vi "Write To Csv.vi"(0 "File Path":path, 5 "StringArray":string[](array[string]), 7 "delimiter (Tab)":string, 11 "error in (no error)":errorcluster) -> (4 "String Out":string, 15 "error out":errorcluster)   [LabVIEW 2021, in "CustomSortPath.lvlib"]
doc: "This vi gets the file path , string array and delimiter as input. Writes the data into a .csv file."
uses:
  CustomSortPath.lvlib
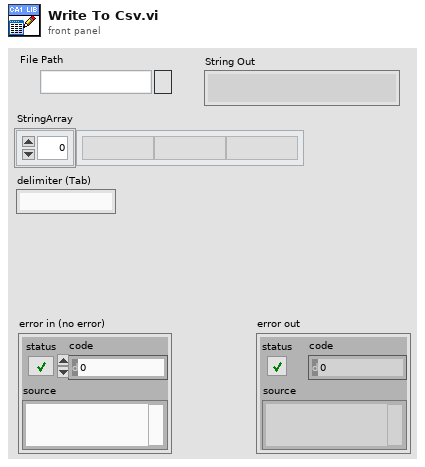
[diagram p1: front panel]
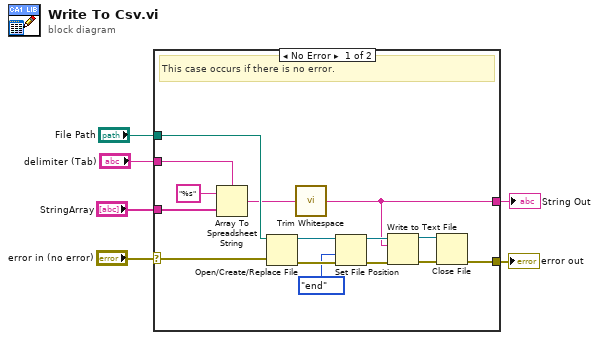
[diagram p0: block diagram]
diagram:
  n1 = case shown="No Error" "error in (no error)" {
    selector: "error in (no error)" -> [w9 w22]
    tunnel: "StringArray" -> [w20 _]
    tunnel: "delimiter (Tab)" -> [w19 _]
    tunnel: "File Path" -> [w18 _]
    tunnel: [w15 w22] -> w3
    tunnel: [w7 _] -> w1
    frame No Error {
      # "This case occurs if there is no error."
      n2 = Array To Spreadsheet String(delimiter (Tab)=w19, array=w20, 3:"%s" ("format string")) -> (spreadsheet string=w8:string)
      n3 = Open/Create/Replace File(file path (use dialog)=w18, error in=w9) -> (refnum out=w12:refnum<file>, error out=w14:errorcluster)  [unwired: 4 in, 1 out]
      n4 = call <vilib>:"Trim Whitespace.vi"("string"=w8) -> ("trimmed string"=w7:string)  [unwired: 1 in]
      n5 = Set File Position(refnum=w12, from (0:start)=enum16{"start", "end", "current"}."end", error in=w14) -> (refnum out=w10:refnum<file>, error out=w13:errorcluster)  [unwired: 1 in]
      n6 = Write to Text File(file (use dialog)=w10, text=w7, error in=w13) -> (refnum out=w16:refnum<file>, error out=w17:errorcluster)  [unwired: 1 in, 1 out]
      n7 = Close File(refnum=w16, error in=w17) -> (error out=w15:errorcluster)  [unwired: 1 out]
    }
    frame Error {
      # "This case occurs if there is any error."
    }
  }
  "error out" <- w3
  "String Out" <- w1
